vi "TOP_LEVEL.vi"() -> ()   [LabVIEW 2013]
panel:
  in  "Dissable initial checks for loop testing":bool
  out "ERRORS":i32
  out "String 2":string
  out "Test Cycles":i32
  out "String":string
  in  "stop":bool=TRUE
  in  "ERROR WIN TEST":bool=TRUE
  in  "SPEED BITS TEST":bool
  out "Boolean 2":bool
  out "Boolean":bool
  out "Array":bool[](array[boolean])
  in  "WRITE TO FILE?":bool
  in  "CHOPPER SERIAL NUMBER":i32=69 min=0 max=99 step=1
  in  "OPTICAL IO TESTS":bool
  in  "DATA VETO TESTS":bool=TRUE
  in  "MP SYNC TESTS":bool=TRUE
  in  "SINGLE BIT FUNCTIONS":bool=TRUE
  out "PASS / FAIL":bool
  out "REPORT":string
  in  "CONTROLLER OUTPUTS":bool=TRUE
  # "INPUT & CONTROL PANEL"
  # "OUTPUT PANEL"
  # "MODULE IS MOVING TO REFERENCE"
  # "MODULE READY?"
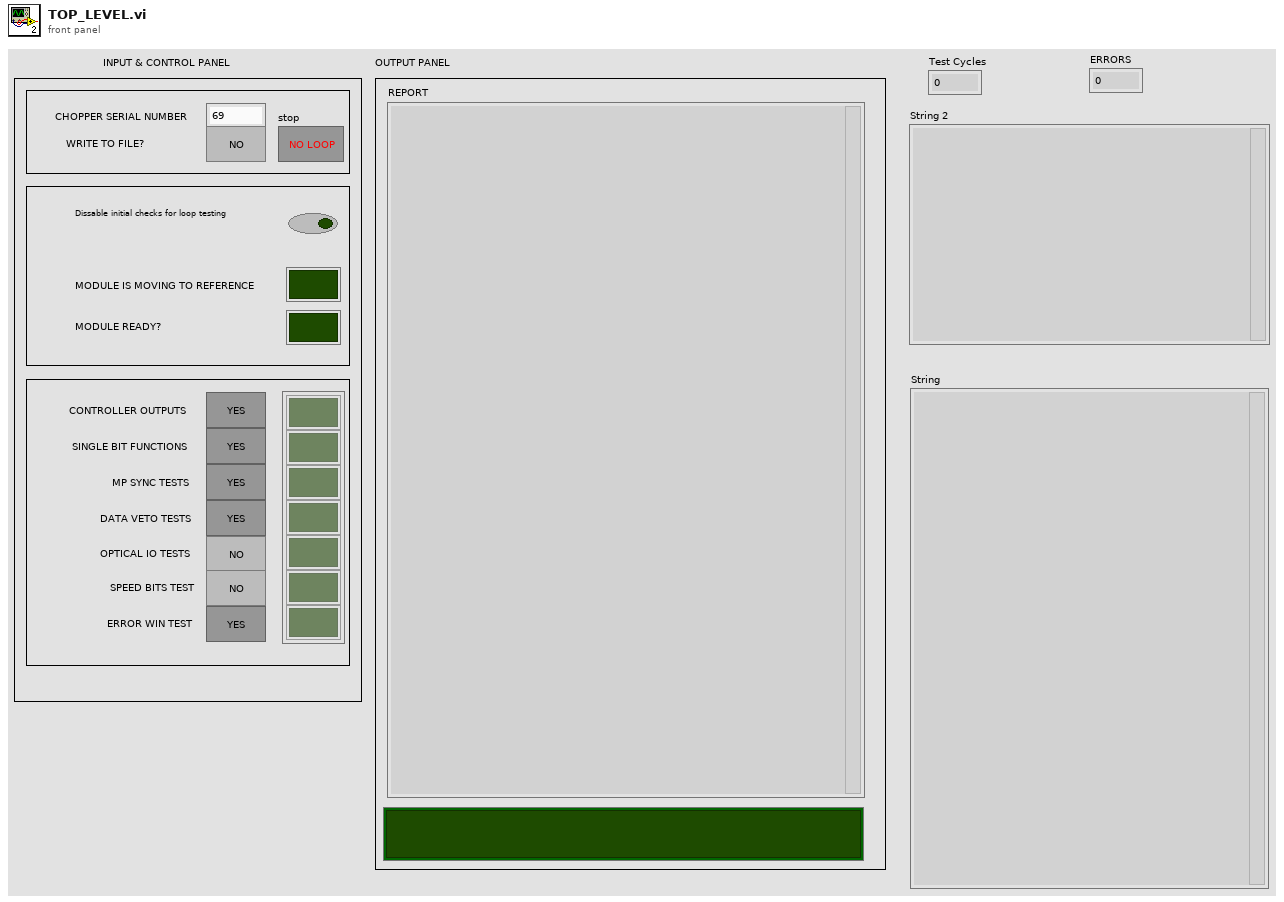
[diagram p1: front panel]
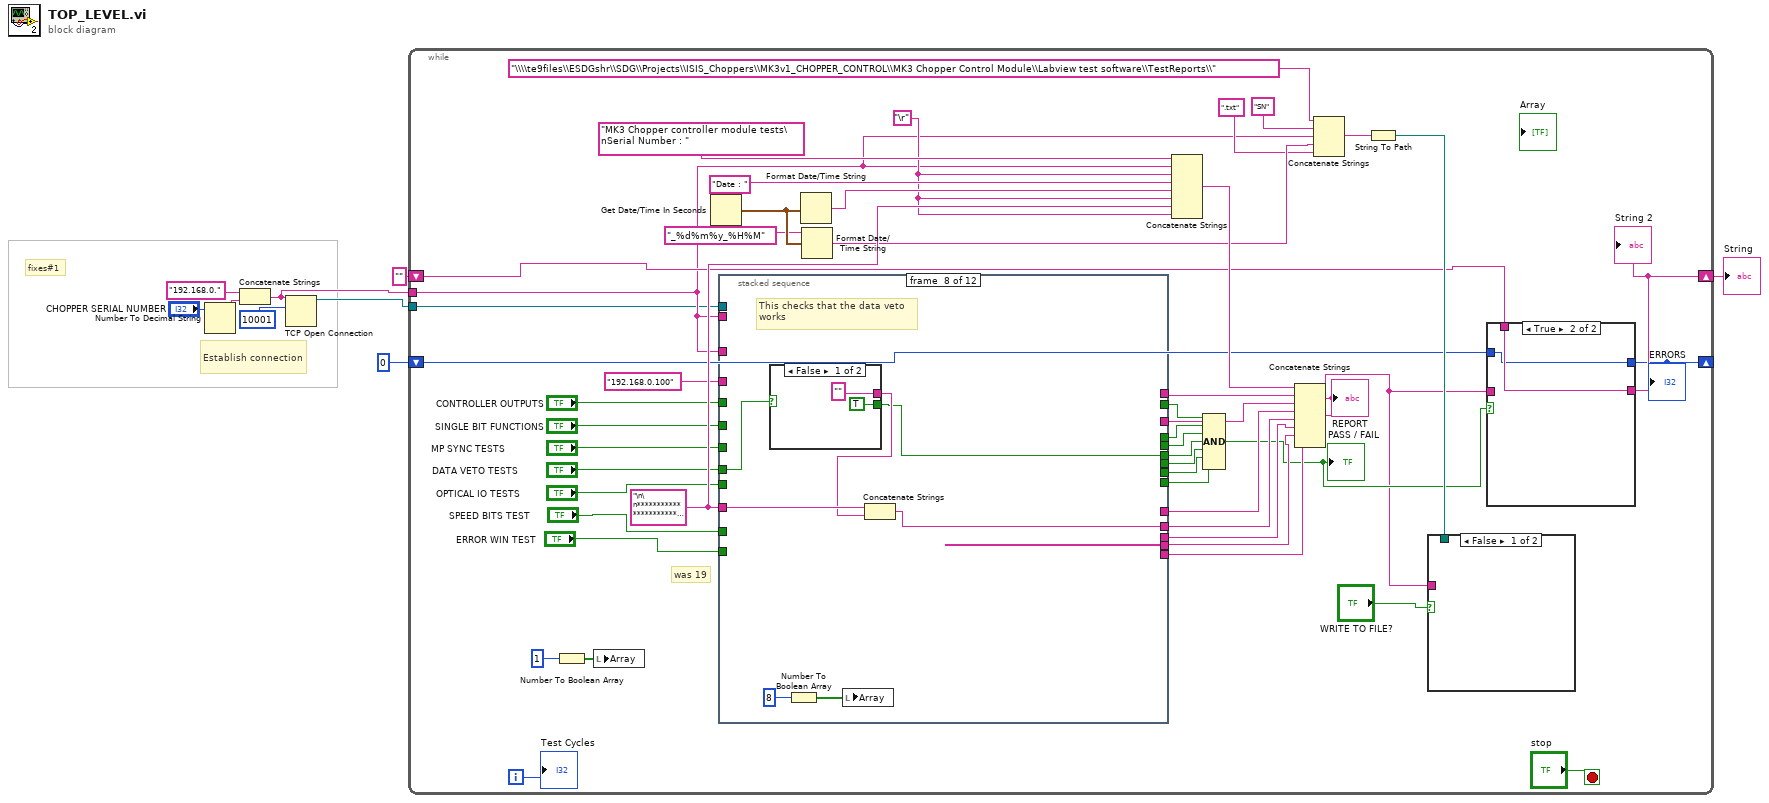
[diagram p0: block diagram]
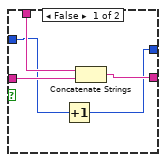
[diagram p2: hidden frame]
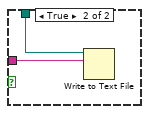
[diagram p3: hidden frame]
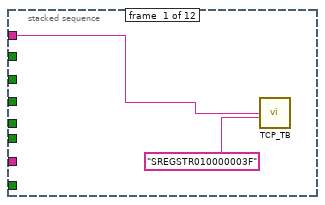
[diagram p4: hidden frame]
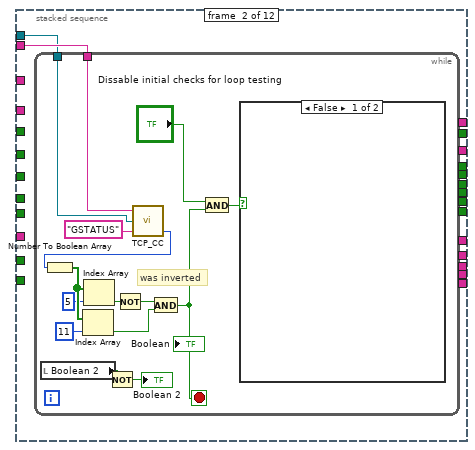
[diagram p5: hidden frame]
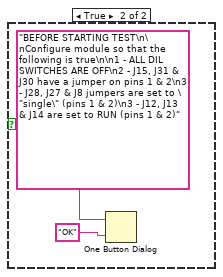
[diagram p6: hidden frame]
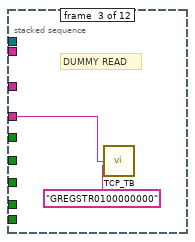
[diagram p7: hidden frame]
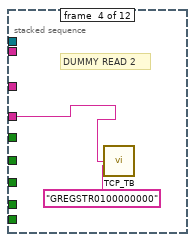
[diagram p8: hidden frame]
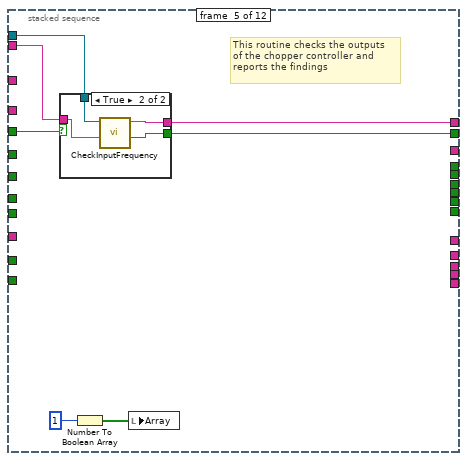
[diagram p9: hidden frame]
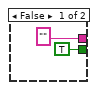
[diagram p10: hidden frame]
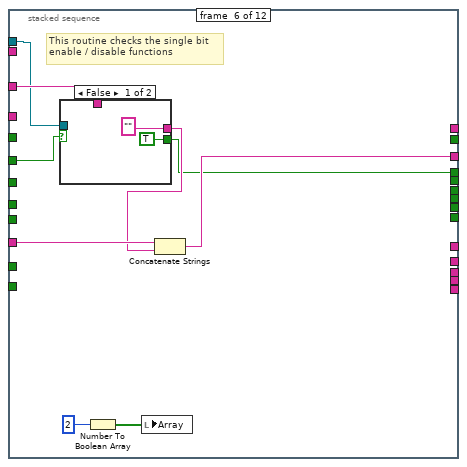
[diagram p11: hidden frame]
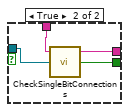
[diagram p12: hidden frame]
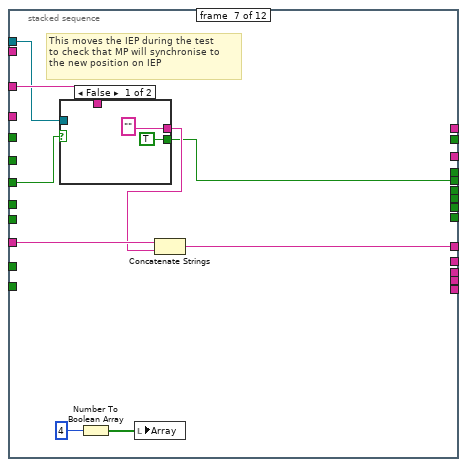
[diagram p13: hidden frame]
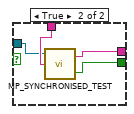
[diagram p14: hidden frame]
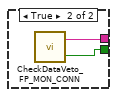
[diagram p15: hidden frame]
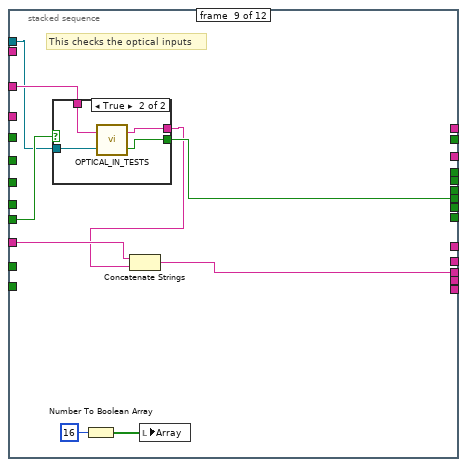
[diagram p16: hidden frame]
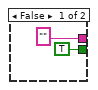
[diagram p17: hidden frame]
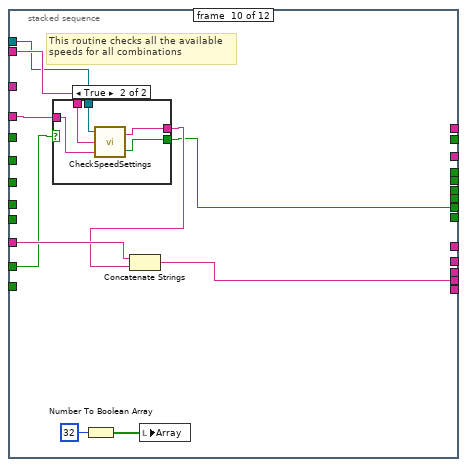
[diagram p18: hidden frame]
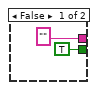
[diagram p19: hidden frame]
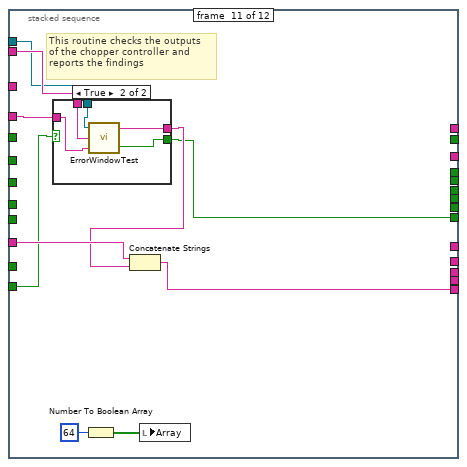
[diagram p20: hidden frame]
diagram:
  # "fixes#1"
  # "Establish connection"
  n1 = Number To Decimal String(number="CHOPPER SERIAL NUMBER") -> (decimal integer string=w3:string)  [unwired: 1 in]
  n2 = Concatenate Strings("192.168.0." ("TB IP ADDRESS"), w3) -> (w2:string)
  n3 = TCP Open Connection(address=w2, remote port or service name=u16 10001 ("remote port")) -> (connection ID=w1:refnum<k5>)  [unwired: 3 in, 1 out]
  n4 = while {
    shift-right: [w24] -> w8
    shift-left: "" -> [w23]
    shift-right: [w19] -> _
    shift-left: 0 -> [w20]
    tunnel: w2 -> [w11]
    tunnel: w1 -> [w10]
    i -> [w21]
    stop <- "stop" stop-if-true
    w40 = "\r"
    w41 = "\n\n**********************************************\n\n"
    # "was 19"
    n5 = Number To Boolean Array(number=1) -> (Boolean array=w32:bool[])
    n6 = local write "Array"(w32) -> ()
    n7 = Get Date/Time In Seconds() -> (seconds since 1Jan1904=w44:timestamp)
    n8 = stacked-sequence {
      tunnel: "CONTROLLER OUTPUTS" -> [_ _ _ _ w99 _ _ _ _ _ _ _]
      tunnel: [_ _ _ _ w98 _ _ _ _ _ _ _] -> w58
      tunnel: [_ _ _ _ w97 _ _ _ _ _ _ _] -> w57
      tunnel: w41 -> [_ _ _ _ _ w114 w129 w142 w152 w171 w188 _]
      tunnel: "SINGLE BIT FUNCTIONS" -> [_ _ _ _ _ w112 _ _ _ _ _ _]
      tunnel: [_ _ _ _ _ w111 _ _ _ _ _ _] -> w56
      tunnel: [_ _ _ _ _ w110 _ _ _ _ _ _] -> w55
      tunnel: w11 -> [_ _ _ _ _ w109 w127 _ w154 _ _ _]
      tunnel: [_ _ _ _ _ _ w126 _ _ _ _ _] -> w54
      tunnel: [_ _ _ _ _ _ w125 _ _ _ _ _] -> w53
      tunnel: "MP SYNC TESTS" -> [_ _ _ _ _ _ w124 _ _ _ _ _]
      tunnel: [_ _ _ _ _ _ _ w140 _ _ _ _] -> w52
      tunnel: [_ _ _ _ _ _ _ w139 _ _ _ _] -> w51
      tunnel: "DATA VETO TESTS" -> [_ _ _ _ _ _ _ w138 _ _ _ _]
      tunnel: [_ _ _ _ _ _ _ _ w153 _ _ _] -> w50
      tunnel: [_ _ _ _ _ _ _ _ w155 _ _ _] -> w49
      tunnel: "OPTICAL IO TESTS" -> [_ _ _ _ _ _ _ _ w150 _ _ _]
      tunnel: [_ _ _ _ _ _ _ _ _ w167 _ _] -> w31
      tunnel: [_ _ _ _ _ _ _ _ _ w166 _ _] -> w30
      tunnel: "SPEED BITS TEST" -> [_ _ _ _ _ _ _ _ _ w165 _ _]
      tunnel: "192.168.0.100" ("IP ADDRESS") -> [w68 _ w89 w91 _ _ _ _ _ w164 w184 _]
      tunnel: w11 -> [_ w71 _ _ w94 _ _ _ _ w163 w183 _]
      tunnel: [_ _ _ _ _ _ _ _ _ _ w182 _] -> w28
      tunnel: [_ _ _ _ _ _ _ _ _ _ w181 _] -> w27
      tunnel: "ERROR WIN TEST" -> [_ _ _ _ _ _ _ _ _ _ w180 _]
      tunnel: w10 -> [_ w70 _ _ w93 w106 w121 _ w147 w162 w179 _]
      frame #0 {
        n9 = call "TCP_TB.vi"("IP ADDRESS"=w68, "COMMAND"="SREGSTR010000003F") -> ()  [unwired: 4 in, 3 out]
      }
      frame #1 {
        n10 = while {
          tunnel: w71 -> [w85]
          tunnel: w70 -> [w72]
          stop <- w75 stop-if-true
          # "was inverted"
          n11 = local read "Boolean 2"() -> (w78:bool)
          n12 = Not(x=w78) -> (.not. x?=→"Boolean 2":bool)
          n13 = call "TCP_CC.vi"("COMMAND"="GSTATUS", "connection ID"=w72, "IP ADDRESS"=w85) -> ("number"=w84:u32)  [unwired: 2 out]
          n14 = Number To Boolean Array(number=w84) -> (Boolean array=w83:bool[])
          n15 = Index Array(array=w83, index=11) -> (element=w80:bool)
          n16 = Index Array(array=w83, index=5) -> (element=w77:bool)
          n17 = Not(x=w77) -> (.not. x?=w73:bool)
          n18 = And(x=w73, y=w80) -> (x .and. y?=w75:bool)
          "Boolean" <- w75
          n19 = And(x="Dissable initial checks for loop testing", y=w75) -> (x .and. y?=w76:bool)
          n20 = case shown="False" w76 {
            frame False {
            }
            frame True {
              n21 = One Button Dialog(message="BEFORE STARTING TEST\n\nConfigure module so that the following is true\n\n1 - ALL DIL SWITCHES ARE OFF\n2 - J15, J31 & J30 have a jumper on pins 1 & 2\n3 - J28, J27 & J8 jumpers are set to \"single\" (pins 1 & 2)\n3 - J12, J13 & J14 are set to RUN (pins 1 & 2)", button name ("OK")="OK") -> ()  [unwired: 1 out]
            }
          }
        }
      }
      frame #2 {
        # "DUMMY READ"
        n22 = call "TCP_TB.vi"("IP ADDRESS"=w89, "COMMAND"="GREGSTR0100000000") -> ()  [unwired: 4 in, 3 out]
      }
      frame #3 {
        # "DUMMY READ 2"
        n23 = call "TCP_TB.vi"("IP ADDRESS"=w91, "COMMAND"="GREGSTR0100000000") -> ()  [unwired: 4 in, 3 out]
      }
      frame #4 {
        # "This routine checks the outputs\nof the chopper controller and\nreports the findings"
        n24 = case shown="True" w99 {
          tunnel: ["" w105] -> w98
          tunnel: [TRUE ("Success") w104] -> w97
          tunnel: w94 -> [_ w103]
          tunnel: w93 -> [_ w102]
          frame False {
          }
          frame True {
            n25 = call "CheckInputFrequency.vi"("IP ADDRESS"=w103, "Connection ID CC"=w102) -> ("Success"=w104:bool, "String"=w105:string)  [unwired: 4 in, 1 out]
          }
        }
        n26 = Number To Boolean Array(number=1) -> (Boolean array=w95:bool[])
        n27 = local write "Array"(w95) -> ()
      }
      frame #5 {
        # "This routine checks the single bit\nenable / disable functions"
        n28 = case shown="False" w112 {
          tunnel: ["" w120] -> w113
          tunnel: [TRUE ("Success") w119] -> w110
          tunnel: w109 -> [_ w118]
          tunnel: w106 -> [_ w117]
          frame False {
          }
          frame True {
            n29 = call "CheckSingleBitConnections.vi"("connection ID CC"=w117, "Chopper Serial Number"=w118) -> ("PASS / FAIL"=w119:bool, "RESULT"=w120:string)  [unwired: 1 in, 1 out]
          }
        }
        n30 = Number To Boolean Array(number=2) -> (Boolean array=w107:bool[])
        n31 = local write "Array"(w107) -> ()
        n32 = Concatenate Strings(w114, w113) -> (w111:string)
      }
      frame #6 {
        # "This moves the IEP during the test\nto check that MP will synchronise to\nthe new position on IEP"
        n33 = case shown="False" w124 {
          tunnel: ["" w135] -> w128
          tunnel: [TRUE ("Success") w134] -> w125
          tunnel: w127 -> [_ w133]
          tunnel: w121 -> [_ w132]
          frame False {
          }
          frame True {
            n34 = call "MP_SYNCHRONISED_TEST.vi"("Chopper Serial Number"=w133, "connection ID CC"=w132) -> ("PASS / FAIL"=w134:bool, "concatenated string"=w135:string)  [unwired: 1 in]
          }
        }
        n35 = Number To Boolean Array(number=4) -> (Boolean array=w122:bool[])
        n36 = local write "Array"(w122) -> ()
        n37 = Concatenate Strings(w129, w128) -> (w126:string)
      }
      frame #7 {
        # "This checks that the data veto\nworks"
        n38 = case shown="False" w138 {
          tunnel: ["" w146] -> w141
          tunnel: [TRUE ("Success") w145] -> w139
          frame False {
          }
          frame True {
            n39 = call "CheckDataVeto_FP_MON_CONN.vi"() -> ("PASS / FAIL"=w145:bool, "concatenated string"=w146:string)  [unwired: 2 in]
          }
        }
        n40 = Number To Boolean Array(number=8) -> (Boolean array=w136:bool[])
        n41 = local write "Array"(w136) -> ()
        n42 = Concatenate Strings(w142, w141) -> (w140:string)
      }
      frame #8 {
        # "This checks the optical inputs"
        n43 = case shown="True" w150 {
          tunnel: ["" w161] -> w151
          tunnel: [TRUE ("Success") w159] -> w155
          tunnel: w154 -> [_ w160]
          tunnel: w147 -> [_ w158]
          frame False {
          }
          frame True {
            n44 = call "OPTICAL_IN_TESTS.vi"("connection ID CC"=w158, "Chopper Serial Number"=w160) -> ("PASS / FAIL"=w159:bool, "concatenated string"=w161:string)
          }
        }
        n45 = Number To Boolean Array(number=16) -> (Boolean array=w148:bool[])
        n46 = Concatenate Strings(w152, w151) -> (w153:string)
        n47 = local write "Array"(w148) -> ()
      }
      frame #9 {
        # "This routine checks all the available\nspeeds for all combinations"
        n48 = case shown="True" w165 {
          tunnel: ["" w177] -> w170
          tunnel: [TRUE ("Success") w176] -> w166
          tunnel: w163 -> [_ w178]
          tunnel: w164 -> [_ w175]
          tunnel: w162 -> [_ w174]
          frame False {
          }
          frame True {
            n49 = call "CheckSpeedSettings.vi"("TB IP ADDRESS"=w175, "CC IP ADDRESS"=w178, "connection ID CC"=w174) -> ("PASS"=w176:bool, "String 2"=w177:string)
          }
        }
        n50 = Number To Boolean Array(number=32) -> (Boolean array=w168:bool[])
        n51 = Concatenate Strings(w171, w170) -> (w167:string)
        n52 = local write "Array"(w168) -> ()
      }
      frame #10 {
        # "This routine checks the outputs\nof the chopper controller and\nreports the findings"
        n53 = case shown="True" w180 {
          tunnel: ["" w195] -> w187
          tunnel: [TRUE ("Success") w194] -> w182
          tunnel: w183 -> [_ w193]
          tunnel: w184 -> [_ w192]
          tunnel: w179 -> [_ w191]
          frame False {
          }
          frame True {
            n54 = call "ErrorWindowTest.vi"("IP ADDRESS 2"=w192, "IP ADDRESS"=w193, "connection ID CC"=w191) -> ("PASS / FAIL"=w194:bool, "REPORT LOG"=w195:string)
          }
        }
        n55 = Number To Boolean Array(number=64) -> (Boolean array=w185:bool[])
        n56 = Concatenate Strings(w188, w187) -> (w181:string)
        n57 = local write "Array"(w185) -> ()
      }
      frame #11 {
        n58 = Number To Boolean Array(number=0) -> (Boolean array=w196:bool[])
        n59 = local write "Array"(w196) -> ()
      }
    }
    n60 = Format Date/Time String(seconds (now)=w44) -> (date/time string=w43:string)  [unwired: 2 in]
    n61 = Format Date/Time String(time format string (%c)="_%d%m%y_%H%M", seconds (now)=w44) -> (date/time string=w38:string)  [unwired: 1 in]
    n62 = Concatenate Strings("MK3 Chopper controller module tests\nSerial Number : " ("Chopper Serial Number"), w11, w40, "Date : " ("Chopper Serial Number"), w43, w40, w41, w40) -> (w47:string)
    n63 = Compound Arithmetic op=AND(w57, w55, w53, w51, w49, w30, w28) -> (w25:bool)
    "PASS / FAIL" <- w25
    n64 = Concatenate Strings(w47, w58, w56, w54, w52, w50, w31, w27) -> (w22:string)
    "REPORT" <- w22
    n65 = Concatenate Strings("\\\\te9files\\ESDGshr\\SDG\\Projects\\ISIS_Choppers\\MK3v1_CHOPPER_CONTROL\\MK3 Chopper Control Module\\Labview test software\\TestReports\\" ("string"), "SN" ("string"), w11, w38, ".txt" ("string")) -> (w37:string)
    n66 = String To Path(string=w37) -> (path=w36:path)
    n67 = case shown="False" "WRITE TO FILE?" {
      tunnel: w36 -> [_ w67]
      tunnel: w22 -> [_ w66]
      frame False {
      }
      frame True {
        n68 = Write to Text File(file (use dialog)=w67, text=w66) -> ()  [unwired: 2 in, 3 out]
      }
    }
    n69 = case shown="True" w25 {
      tunnel: [w63 w65] -> w24
      tunnel: w23 -> [w62 w65]
      tunnel: w22 -> [w61 _]
      tunnel: w20 -> [w60 w64]
      tunnel: [w59 w64] -> w19
      frame False {
        n70 = Increment(x=w60) -> (x+1=w59:i32)
        n71 = Concatenate Strings(w62, w61) -> (w63:string)
      }
      frame True {
      }
    }
    "String 2" <- w24
    "ERRORS" <- w19
    "Test Cycles" <- w21
  }
  "String" <- w8
